vi "SubVI_Search.vi"(6 "Numeric 2":i32, 9 "Silinecek ID":i32, 10 "Kullanıcı Bilgileri":T1 {"Boy" min=1.0 max=2.5 step=0.01; "Yaş" min=10.0 max=100.0}, 11 "Kullanıcı Listesi":T2) -> (2 "Arama Sonucu":string, 3 "Stop(while)":bool)   [LabVIEW 2024]
uses:
  Control 3.ctl
  Documents/LabView Projects/Control 1.ctl
  Control 2_1.ctl
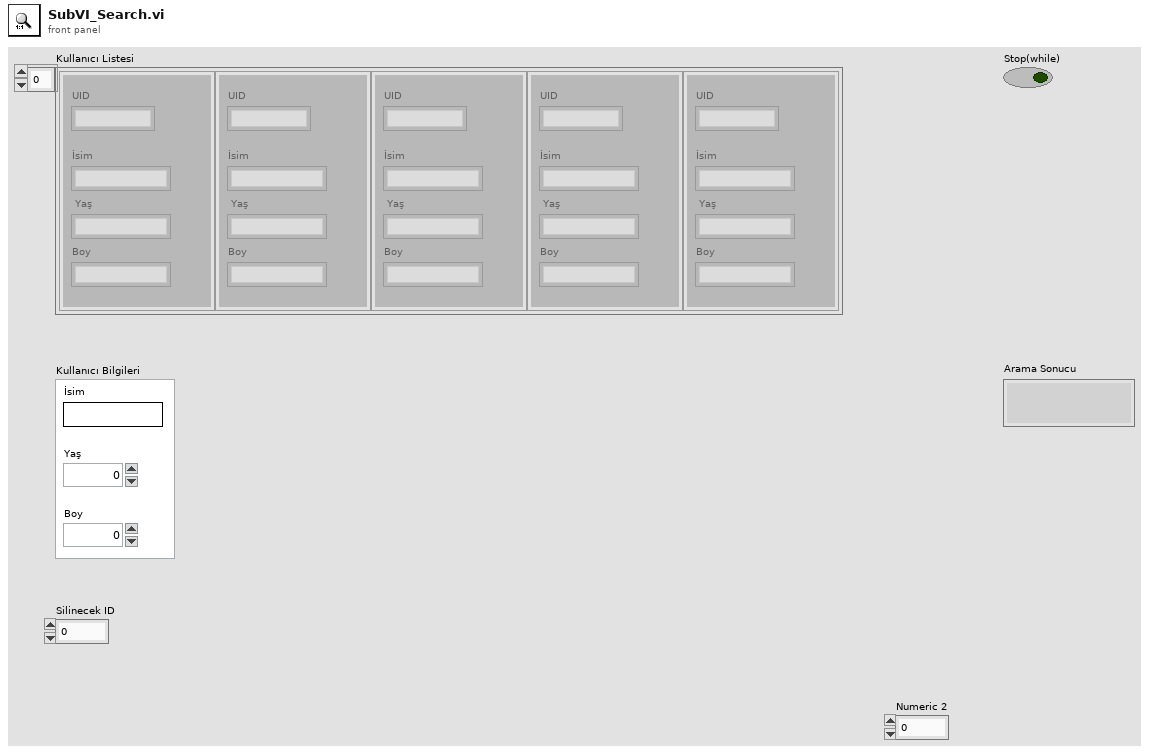
[diagram p1: front panel]
types:
  T1 = typedef "Control 2_1.ctl" = cluster{"İsim":string, "Yaş":dbl, "Boy":dbl}
  T2 = typedef "Control 3.ctl" = T3[]
  T3 = typedef "Control 1.ctl" = cluster{"UID":string, "İsim":string, " Yaş":string, "Boy":string}
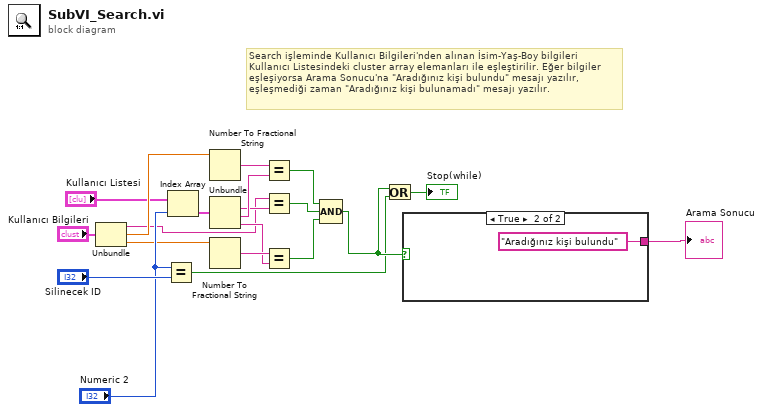
[diagram p0: block diagram]
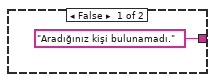
[diagram p2: hidden frame]
diagram:
  # "Search işleminde Kullanıcı Bilgileri'nden alınan İsim-Yaş-Boy bilgileri \nKullanıcı Listesindeki cluster array elemanları ile eşleştirilir. Eğer bilgiler \neşleşiyorsa Arama Sonucu'na \"Aradığınız kişi bulundu\" mesajı yazılır, \neşleşmediği zaman \"Aradığınız kişi bulunamadı\" mesajı yazılır."
  n1 = Unbundle("Kullanıcı Bilgileri") -> ("İsim"=w3:string, "Yaş"=w6:dbl, "Boy"=w7:dbl)
  n2 = Equal?(x="Numeric 2", y="Silinecek ID") -> (x = y?=w14:bool)
  n3 = Index Array(array="Kullanıcı Listesi", index="Numeric 2") -> (element=w2:T3)
  n4 = Number To Fractional String(number=w6) -> (F-format string=w8:string)  [unwired: 3 in]
  n5 = Unbundle(w2) -> ("İsim"=w4:string, "Yaş"=w9:string, "Boy"=w10:string)  [unwired: 1 out]
  n6 = Number To Fractional String(number=w7) -> (F-format string=w11:string)  [unwired: 3 in]
  n7 = Equal?(x=w8, y=w9) -> (x = y?=w17:bool)
  n8 = Equal?(x=w3, y=w4) -> (x = y?=w18:bool)
  n9 = Equal?(x=w11, y=w10) -> (x = y?=w19:bool)
  n10 = Compound Arithmetic op=AND(w17, w18, w19) -> (w20:bool)
  n11 = Or(x=w20, y=w14) -> (x .or. y?=→"Stop(while)":bool)
  n12 = case shown="True" w20 {
    tunnel: ["Aradığınız kişi bulunamadı." "Aradığınız kişi bulundu"] -> w16
    frame False {
    }
    frame True {
    }
  }
  "Arama Sonucu" <- w16
